vi "Set Cluster Element by Name__ogtk_TS.vi"(8 "error in (no error)":errorcluster, 9 "Element Name (\"\": New Element Data Name)":string, 10 "New Element Value":variant, 11 "Cluster":variant) -> (0 "error out":errorcluster, 1 "found?":bool, 3 "VCluster out":variant)   [LabVIEW 2011]
doc: "Returns a cluster with element replaced with new element value. If <B>Element name</B> unwired, <B>New Element Value</B> data name is used. Data type of the new element is not checked for compatibility with replaced element."
panel:
  out "Data Name":string
  # "offset.Channel1.Value"
  # "[OpenG VI Tags] ***Do Not Remove***\nSVN Revision = 827\nSVN Revision Date = 2008-04-30 16:06:27 -0700 (Wed, 30 Apr 2008)\nPackage = oglib_lvdata-2.9-1\nDepends = oglib_error-2.0-1"
  # "Set Cluster Element by Name.vi\n\nReturns a cluster with element replaced with new element value. If <B>Element na\n\nPlease visit http://www.OpenG.org to learn about the\nOpen Source LabVIEW software movement.\n\nNOTICE -- YOU MUST LEAVE THIS NOTICE IN PLACE.  PER THE TERMS OF THE LICENSE BELOW, YOU MAY SUBLICENSE THIS SOFTWARE \nIN ANY WAY THAT DOES NOT CONFLICT WITH THIS LICENSE.\n\n### BSD License (http://www.opensource.org/licenses/bsd-license.php) Begin ###\n \nCopyright (c) 2002, Jean-Pierre Drolet <drolet_jp@hotmail.com>\nCopyright (c) 2002-2006, Jim Kring <jim@jimkring.com>\n\nAll rights reserved.\n\nRedistribution and use in source and binary forms, with or without modification, are permitted provided that the following conditions are met:\n\n    * Redistributions of source code must retain the above copyright notice, this list of conditions and the following disclaimer.\n    * Redistributions in binary form must reproduce the above copyright notice, this list of conditions and the following disclaimer in the \n       documentation and/or other materials provided with the distribution.\n    * Neither the name of SciWare, James Kring, Inc., nor the names of its contributors may be used to endorse or promote products derived \n       from this software without specific prior written permission.\n\nTHIS SOFTWARE IS PROVIDED BY THE COPYRIGHT HOLDERS AND CONTRIBUTORS \"AS IS\" AND ANY EXPRESS OR IMPLIED WARRANTIES, \nINCLUDING, BUT NOT LIMITED TO, THE IMPLIED WARRANTIES OF MERCHANTABILITY AND FITNESS FOR A PARTICULAR PURPOSE ARE \nDISCLAIMED. IN NO EVENT SHALL THE COPYRIGHT OWNER OR CONTRIBUTORS BE LIABLE FOR ANY DIRECT, INDIRECT, INCIDENTAL,\n SPECIAL, EXEMPLARY, OR CONSEQUENTIAL DAMAGES (INCLUDING, BUT NOT LIMITED TO, PROCUREMENT OF SUBSTITUTE GOODS OR \nSERVICES; LOSS OF USE, DATA, OR PROFITS; OR BUSINESS INTERRUPTION) HOWEVER CAUSED AND ON ANY THEORY OF LIABILITY, \nWHETHER IN CONTRACT, STRICT LIABILITY, OR TORT (INCLUDING NEGLIGENCE OR OTHERWISE) ARISING IN ANY WAY OUT OF THE USE \nOF THIS SOFTWARE, EVEN IF ADVISED OF THE POSSIBILITY OF SUCH DAMAGE.\n\n### BSD License End ###"
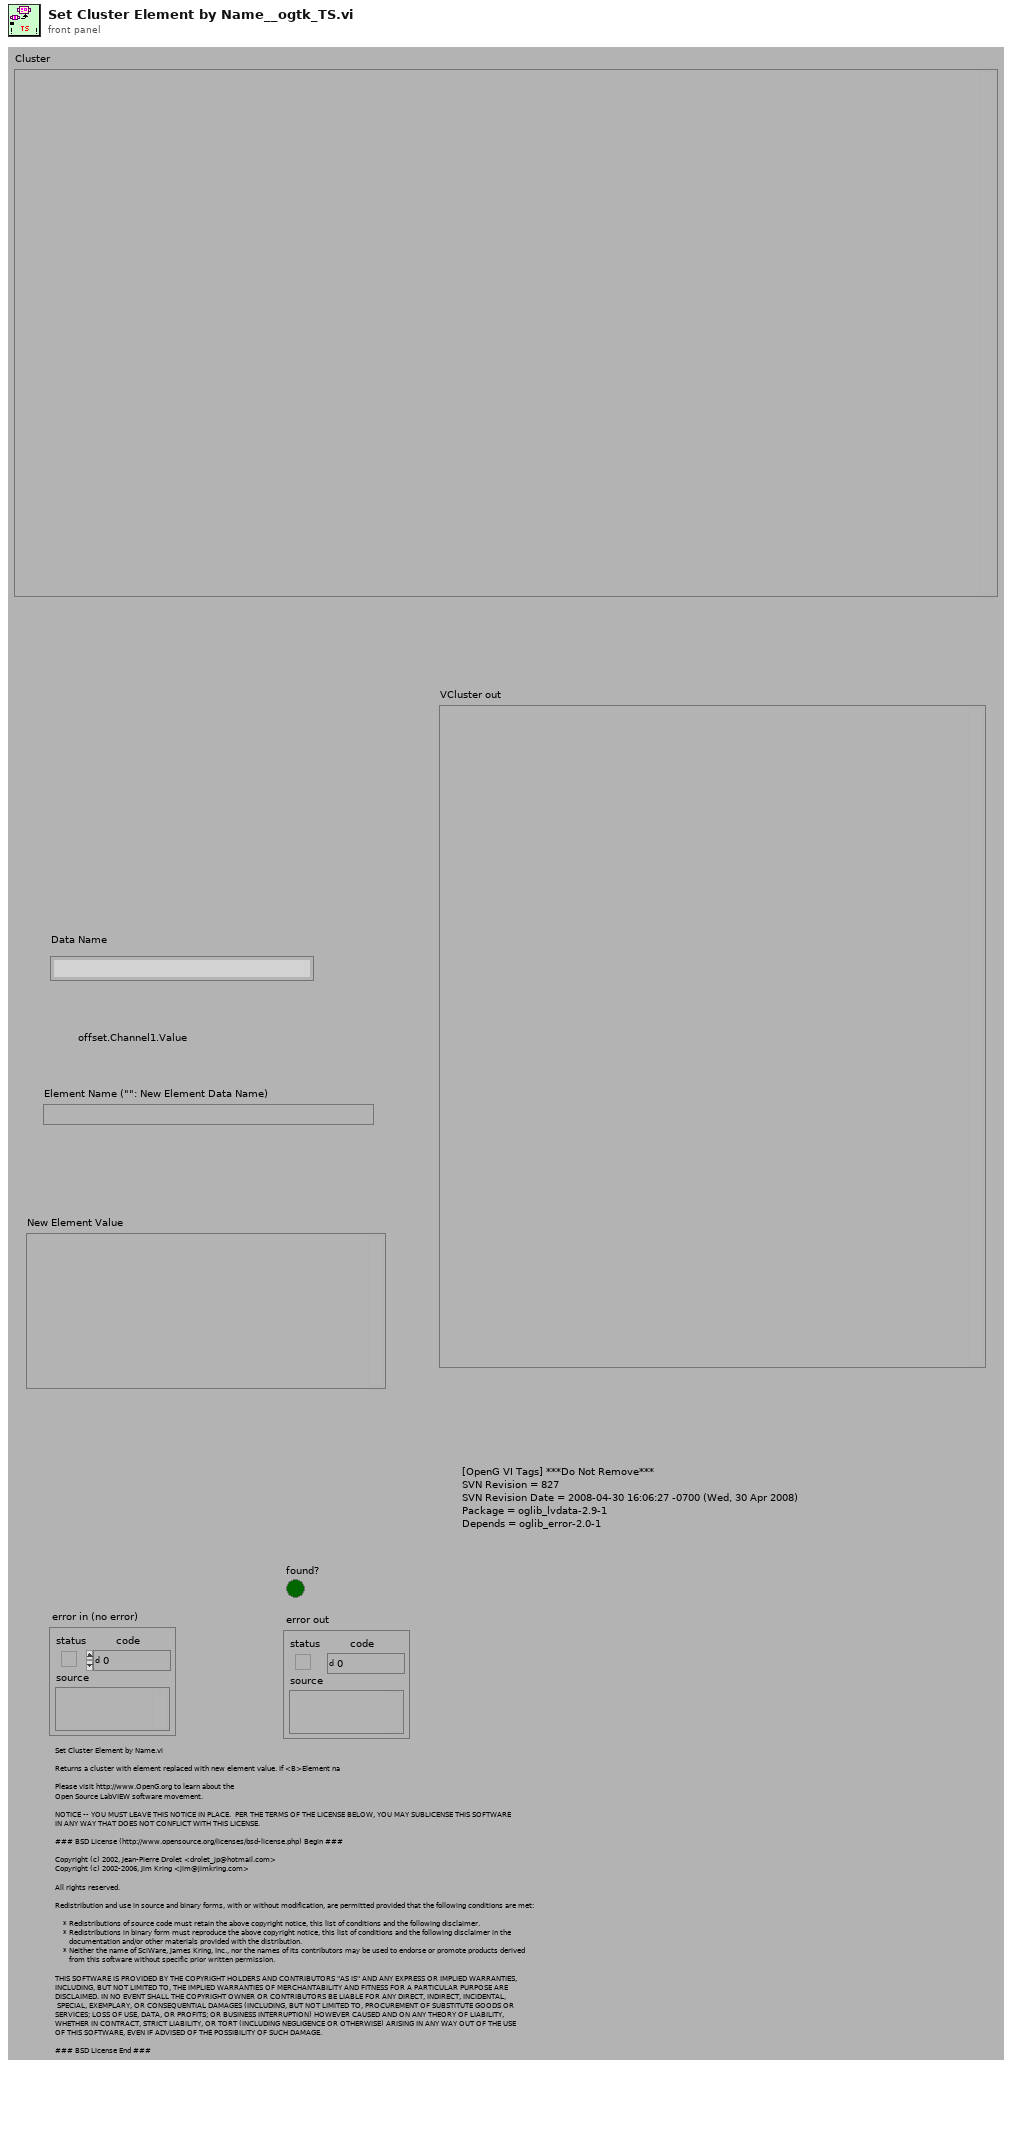
[diagram p1: front panel]
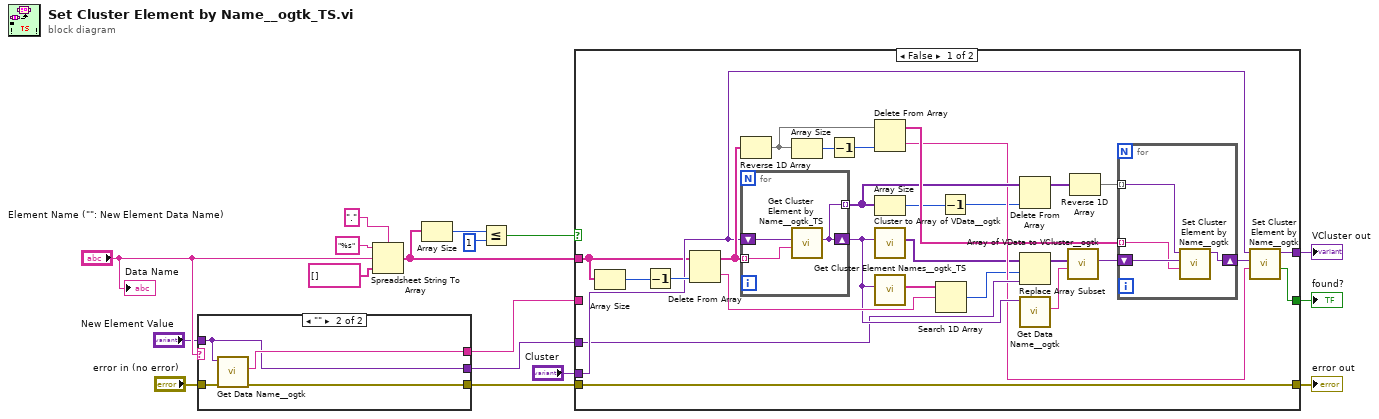
[diagram p0: block diagram]
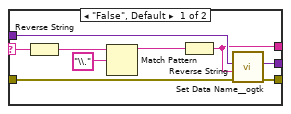
[diagram p2: hidden frame]
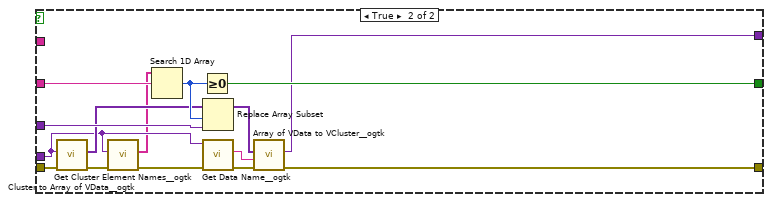
[diagram p3: hidden frame]
diagram:
  n1 = case shown="\"\"" "Element Name (\"\": New Element Data Name)" {
    selector: "Element Name (\"\": New Element Data Name)" -> [w18 _]
    tunnel: "New Element Value" -> [w26 w27]
    tunnel: [w19 w30] -> w9
    tunnel: [w25 w27] -> w14
    tunnel: "error in (no error)" -> [w24 w29]
    tunnel: [w23 w28] -> w17
    frame "False", Default {
      n2 = Reverse String(1:w18) -> (0:w22:string)
      n3 = Match Pattern(string=w22, regular expression="\\.") -> (before substring=w20:string)  [unwired: 1 in, 3 out]
      n4 = Reverse String(1:w20) -> (0:w19:string)
      n5 = call "Set Data Name__ogtk.vi"("error in (no error)"=w24, "Data Name"=w19, "Data"=w26) -> ("error out"=w23:errorcluster, "Renamed Data"=w25:variant)  [unwired: 7 in]
    }
    frame "" {
      n6 = call "Get Data Name__ogtk.vi"("error in (no error)"=w29, "Data"=w27) -> ("error out"=w28:errorcluster, "Data Name"=w30:string)  [unwired: 7 in, 1 out]
    }
  }
  n7 = Spreadsheet String To Array(delimiter (Tab)=".", format string="%s", spreadsheet string="Element Name (\"\": New Element Data Name)", array type (2D Dbl)=string[] []) -> (array=w13:string[])
  n8 = Array Size(array=w13) -> (size(s)=w5:i32)
  n9 = Less Or Equal?(x=w5, y=1) -> (x <= y?=w12:bool)
  n10 = case shown="False" w12 {
    tunnel: w17 -> [w41 w79]
    tunnel: w9 -> [_ w78]
    tunnel: w14 -> [w42 w76]
    tunnel: "Cluster" -> [w45 w70]
    tunnel: [w43 w75] -> w16
    tunnel: [w41 w74] -> w15
    tunnel: [w44 w73] -> w10
    tunnel: w13 -> [w40 _]
    frame False {
      n11 = Array Size(array=w40) -> (size(s)=w46:i32)
      n12 = Decrement(x=w46) -> (x-1=w49:i32)
      n13 = Delete From Array(array=w40, index=w49) -> (deleted portion=w50:string, array with subset deleted=w52:string[])  [unwired: 1 in]
      n14 = Reverse 1D Array(array=w52) -> (reversed array=w57:string[])
      n15 = for {
        tunnel: w52 -> [w65] mode=indexing
        shift-right: [w63] -> w48
        shift-left: w45 -> [w64]
        tunnel: [w63] -> w53 mode=indexing
        n16 = call "Get Cluster Element by Name__ogtk_TS.vi"("Element Name"=w65, "Cluster"=w64) -> ("VElement"=w63:variant)  [unwired: 7 in, 2 out]
      }
      n17 = Array Size(array=w57) -> (size(s)=w37:i32)
      n18 = Decrement(x=w37) -> (x-1=w38:i32)
      n19 = Delete From Array(array=w57, index=w38) -> (deleted portion=w39:string, array with subset deleted=w58:string[])  [unwired: 1 in]
      n20 = Array Size(array=w53) -> (size(s)=w36:i32)
      n21 = call "Cluster to Array of VData__ogtk.vi"("Cluster"=w48) -> ("Array of VData"=w33:variant[])  [unwired: 9 in, 1 out]
      n22 = call "Get Cluster Element Names__ogtk_TS.vi"("Variant"=w48) -> ("Names (Array)"=w32:string[])  [unwired: 9 in, 1 out]
      n23 = Search 1D Array(1D array=w32, element=w50) -> (index of element=w34:i32)  [unwired: 1 in]
      n24 = Decrement(x=w36) -> (x-1=w35:i32)
      n25 = Delete From Array(array=w53, index=w35) -> (array with subset deleted=w54:variant[])  [unwired: 1 in, 1 out]
      n26 = Replace Array Subset(array=w33, new element=w42, index=w34) -> (w47:variant[])
      n27 = call "Get Data Name__ogtk.vi"("Data"=w48) -> ("Data Name"=w31:string)  [unwired: 8 in, 2 out]
      n28 = call "Array of VData to VCluster__ogtk.vi"("Cluster Name"=w31, "Array"=w47) -> ("VCluster"=w51:variant)  [unwired: 8 in, 1 out]
      n29 = Reverse 1D Array(array=w54) -> (reversed array=w55:variant[])
      n30 = for {
        tunnel: w55 -> [w61] mode=indexing
        shift-right: [w60] -> w56
        shift-left: w51 -> [w62]
        tunnel: w58 -> [w59] mode=indexing
        n31 = call "Set Cluster Element by Name__ogtk.vi"("Element Name (\"\": New Element Data Name)"=w59, "New Element Value"=w62, "Cluster"=w61) -> ("VCluster out"=w60:variant)  [unwired: 6 in, 2 out]
      }
      n32 = call "Set Cluster Element by Name__ogtk.vi"("Element Name (\"\": New Element Data Name)"=w39, "New Element Value"=w56, "Cluster"=w45) -> ("found?"=w43:bool, "VCluster out"=w44:variant)  [unwired: 6 in, 1 out]
    }
    frame True {
      n33 = call "Cluster to Array of VData__ogtk.vi"("error in (no error)"=w79, "Cluster"=w70) -> ("error out"=w68:errorcluster, "Array of VData"=w71:variant[])  [unwired: 8 in]
      n34 = call "Get Cluster Element Names__ogtk.vi"("error in (no error)"=w68, "Cluster"=w70) -> ("error out"=w67:errorcluster, "Element Names"=w69:string[])  [unwired: 8 in]
      n35 = Search 1D Array(1D array=w69, element=w78) -> (index of element=w80:i32)  [unwired: 1 in]
      n36 = Greater Or Equal To 0?(x=w80) -> (x >= 0?=w75:bool)
      n37 = Replace Array Subset(array=w71, new element=w76, index=w80) -> (w72:variant[])
      n38 = call "Get Data Name__ogtk.vi"("error in (no error)"=w67, "Data"=w70) -> ("error out"=w77:errorcluster, "Data Name"=w66:string)  [unwired: 7 in, 1 out]
      n39 = call "Array of VData to VCluster__ogtk.vi"("error in (no error)"=w77, "Cluster Name"=w66, "Array"=w72) -> ("error out"=w74:errorcluster, "VCluster"=w73:variant)  [unwired: 7 in]
    }
  }
  "VCluster out" <- w10
  "found?" <- w16
  "error out" <- w15
  "Data Name" <- "Element Name (\"\": New Element Data Name)"
